vi "OAT Prepare Resample Data.vi"(11 "Array":waveform(dbl)[](array[waveform])) -> (0 "channel count":i32, 1 "signal len":i32, 2 "fs":dbl format="%.2f", 3 "Y":dbl[](array[numeric]) format="%.2f", 5 "elapsed length":dbl)   [LabVIEW 2017, in "SoundVib_Resampling.lvlib"]
uses:
  <vilib>/addons/Sound and Vibration/Order Analysis/Resample Order Tracking/SoundVib_Resampling.lvlib
  <vilib>/Waveform/WDTOps.llb/WDT Number of Waveform Samples DBL.vi
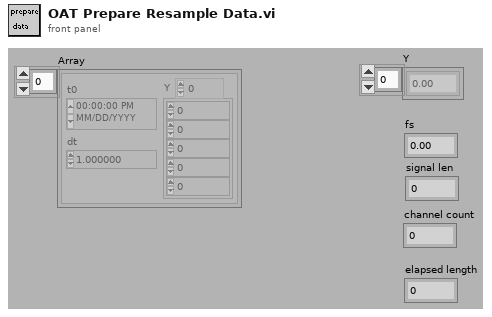
[diagram p1: front panel]
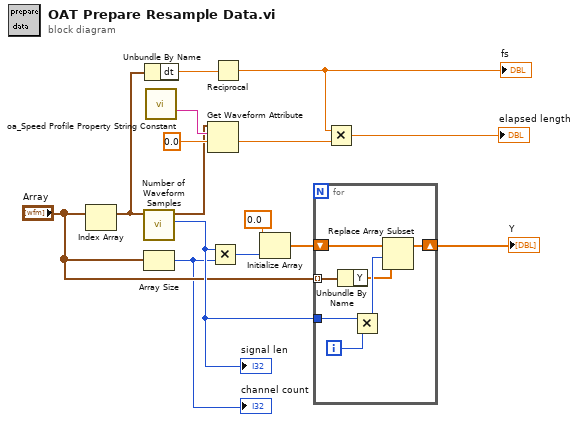
[diagram p0: block diagram]
diagram:
  n1 = Index Array(array="Array") -> (element=w6:waveform(dbl))  [unwired: 1 in]
  n2 = call-poly <vilib>:"Number of Waveform Samples.vi"("waveform in"=w6) -> ("number of samples"=w12:i32, "waveform out"=w1:waveform(dbl))  [unwired: 8 in, 1 out]
  "signal len" <- w12
  n3 = Array Size(array="Array") -> (size(s)=w8:i32)
  "channel count" <- w8
  n4 = Unbundle By Name(w6) -> ("dt"=w9:dbl)
  n5 = call <vilib>:"oa_Speed Profile Property String Constant.vi"() -> ("elapsed time"=w7:string)  [unwired: 12 in, 3 out]
  n6 = Get Waveform Attribute(5:0.0, 6:w7, 7:w1) -> (1:w4:dbl)  [unwired: 1 in, 3 out]
  n7 = Multiply(x=w12, y=w8) -> (x*y=w15:i32)
  n8 = Reciprocal(x=w9) -> (1/x=w3:dbl)
  "fs" <- w3
  n9 = Initialize Array(0.0 ("element"), w15) -> (w13:dbl[])
  n10 = for {
    shift-right: [w16] -> w10
    shift-left: w13 -> [w22]
    tunnel: w12 -> [w20]
    tunnel: "Array" -> [w18] mode=indexing
    i -> [w21]
    n11 = Unbundle By Name(w18) -> ("Y"=w17:dbl[])
    n12 = Multiply(x=w20, y=w21) -> (x*y=w19:i32)
    n13 = Replace Array Subset(array=w22, new element=w17, index=w19) -> (w16:dbl[])
  }
  "Y" <- w10
  n14 = Multiply(x=w3, y=w4) -> (x*y=→"elapsed length":dbl)
